vi "on-off controller sensor 1.vi"(4 "State":i16, 5 "Time":dbl format="%.2f", 6 "Sensor Values":dbl[](array[numeric]), 7 "Set Points":dbl[](array[numeric])) -> (0 "required data":T1={"Set Point names"=["off value", "on value", "minimum target", "maximum target"], "required number of setpoints"=4, "required number of sensors"=1, "Sensor names"=["sensor"]}, 3 "output value":dbl)   [LabVIEW 2019]
panel:
  # "Enter the correct information for this control code in the required data structure below. Then make the current value default by right clicking on the border of the data structure. Select \"data operations\" and then select \"make current value default\". These values will be displayed by process controller."
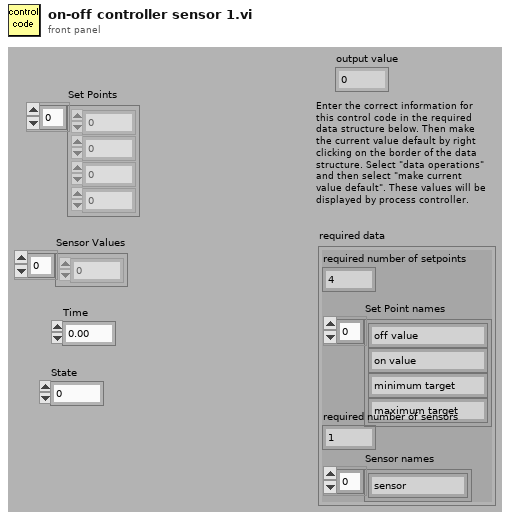
[diagram p1: front panel]
types:
  T1 = cluster{"Set Point names":string[], "required number of setpoints":u8, "required number of sensors":u8, "Sensor names":string[]}
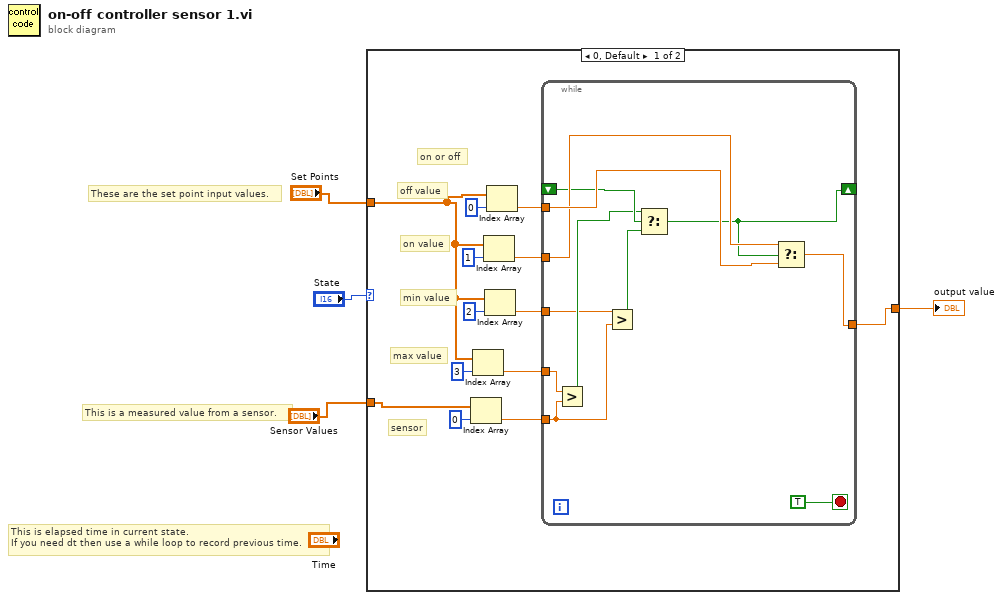
[diagram p0: block diagram]
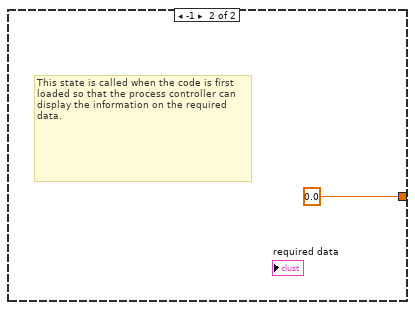
[diagram p2: hidden frame]
diagram:
  # "These are the set point input values."
  # "This is a measured value from a sensor."
  # "This is elapsed time in current state.\nIf you need dt then use a while loop to record previous time."
  n1 = case shown="0, Default" "State" {
    tunnel: [w11 0.0 ("fraction on")] -> w3
    tunnel: "Set Points" -> [w6 _]
    tunnel: "Sensor Values" -> [w9 _]
    frame 0, Default {
      # "on value"
      # "on or off"
      # "sensor"
      # "min value"
      # "max value"
      # "off value"
      n2 = Index Array(array=w9, index=0) -> (element=w8:dbl)
      n3 = Index Array(array=w6, index=3) -> (element=w14:dbl)
      n4 = Index Array(array=w6, index=1) -> (element=w12:dbl)
      n5 = Index Array(array=w6, index=2) -> (element=w16:dbl)
      n6 = Index Array(array=w6, index=0) -> (element=w5:dbl)
      n7 = while {
        tunnel: w16 -> [w20]
        tunnel: w14 -> [w27]
        tunnel: w12 -> [w25]
        tunnel: [w24] -> w11
        tunnel: w8 -> [w19]
        tunnel: w5 -> [w26]
        shift-right: [w21] -> _
        shift-left: _ -> [w23]
        stop <- TRUE stop-if-true
        n8 = Greater?(x=w27, y=w19) -> (0:w22:bool)
        n9 = Greater?(x=w20, y=w19) -> (0:w18:bool)
        n10 = Select(t=w22, s=w23, f=w18) -> (s? t:f=w21:bool)
        n11 = Select(t=w25, s=w21, f=w26) -> (s? t:f=w24:dbl)
      }
    }
    frame -1 {
      # "This state is called when the code is first loaded so that the process controller can display the information on the required data."
    }
  }
  "output value" <- w3
